vi "GetGlobalVisFromProject.vi"() -> ()   [LabVIEW 2020]
panel:
  out "Global Variables in Active Project":string
  # "This tool is used for documenting the global variables in a project.\n\n- Open the prject you want to document\n- Run the VI\n- Check the output in markdown format"
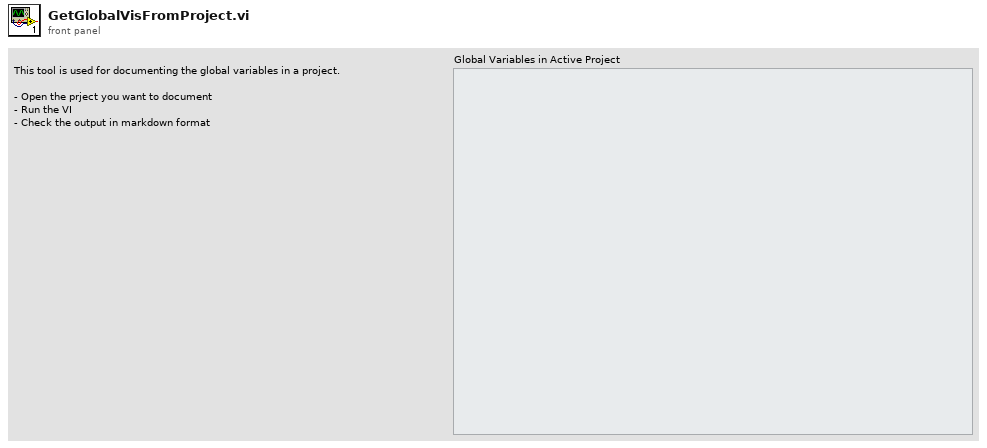
[diagram p1: front panel]
types:
  T1 = enum32{"invalid VI type", "Standard VI", "Control VI", "Global VI", "Polymorphic VI", "Configuration VI", "SubSystem", "Facade VI", "Method VI", "Statechart Diagram VI"}
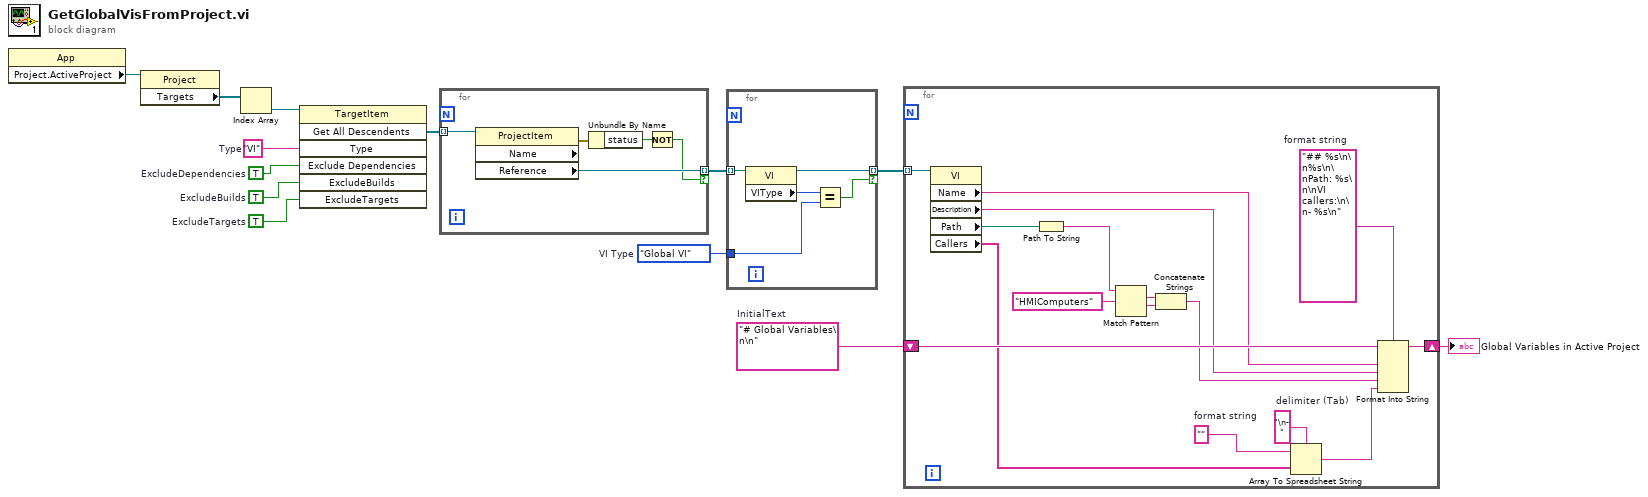
[diagram p0: block diagram]
diagram:
  w2 = "# Global Variables\n\n"  # InitialText
  w4 = T1."Global VI"  # VI Type
  w7 = "VI"  # Type
  w8 = TRUE  # ExcludeTargets
  w9 = TRUE  # ExcludeBuilds
  w10 = TRUE  # ExcludeDependencies
  n1 = property class="App"() -> ("Project.ActiveProject"=w12:refnum<vi>)  [unwired: 2 in, 2 out]
  n2 = property class="Project"(reference=w12) -> ("Targets"=w13:refnum<vi>[])  [unwired: 1 in, 2 out]
  n3 = Index Array(array=w13) -> (element=w11:refnum<vi>)  [unwired: 1 in]
  n4 = invoke class="TargetItem" method="Get All Descendents"(reference=w11, "Type"=w7, "Exclude Dependencies"=w10, "ExcludeBuilds"=w9, "ExcludeTargets"=w8) -> ("All Descendents"=w6:refnum<vi>[])  [unwired: 2 in, 6 out]
  n5 = for {
    tunnel: w6 -> [w18] mode=indexing
    tunnel: [w17] -> w5 mode=indexing if=w14
    n6 = property class="ProjectItem" props=["Name", "Reference"](reference=w18) -> (error out=w16:errorcluster, "Reference"=w17:refnum<vi>)  [unwired: 1 in, 2 out]
    n7 = Unbundle By Name(w16) -> ("status"=w15:bool)
    n8 = Not(x=w15) -> (.not. x?=w14:bool)
  }
  n9 = for {
    tunnel: w5 -> [w23] mode=indexing
    tunnel: [w19] -> w3 mode=indexing if=w20
    tunnel: w4 -> [w21]
    n10 = property class="VI"(reference=w23) -> (reference out=w19:refnum<vi>, "VIType"=w22:T1)  [unwired: 1 in, 1 out]
    n11 = Equal?(x=w22, y=w21) -> (x = y?=w20:bool)
  }
  n12 = for {
    tunnel: w3 -> [w39] mode=indexing
    shift-right: [w37] -> w1
    shift-left: w2 -> [w38]
    w32 = ""  # format string
    w33 = "\n- "  # delimiter (Tab)
    w36 = "## %s\n\n%s\n\nPath: %s\n\nVI callers:\n\n- %s\n"  # format string
    n13 = property class="VI"(reference=w39) -> ("Name"=w35:string, "Description"=w24:string, "Path"=w26:path, "Callers"=w34:string[])  [unwired: 1 in, 2 out]
    n14 = Path To String(path=w26) -> (string=w30:string)
    n15 = Match Pattern(string=w30, regular expression="HMIComputers") -> (match substring=w28:string, after substring=w27:string)  [unwired: 1 in, 2 out]
    n16 = Concatenate Strings(w28, w27) -> (w25:string)
    n17 = Array To Spreadsheet String(delimiter (Tab)=w33, array=w34, 3:w32) -> (spreadsheet string=w31:string)
    n18 = Format Into String(format string=w36, initial string=w38, w35, w24, w25, w31) -> (resulting string=w37:string)  [unwired: 1 in, 1 out]
  }
  "Global Variables in Active Project" <- w1
